vi "Main.vi"() -> ()   [LabVIEW 2014]
uses:
  bus_button.xctl
  VESA_Status.ctl
  Main_status.ctl
  <vilib>/Instr/_visa.llb/VISA Configure Serial Port (Instr).vi
  <vilib>/Instr/_visa.llb/VISA Serial Break (Instr).vi
panel:
  out "수신문자열(TEXT)":string
  in  "OUTPUT PULSE MODE":enum16{"uPPM(400Hz)", "PPM(40Hz)"}(ring)=enum."PPM(40Hz)"
  in  "서보제어":T1(array[cluster])=[{"리모트\nON/OFF"=TRUE, "PPM PULSE (ms)"=1500}, {"리모트\nON/OFF"=FALSE, "PPM PULSE (ms)"=1500}, {"리모트\nON/OFF"=FALSE, "PPM PULSE (ms)"=1500}] {"PPM PULSE (ms)" min=1000 max=2000 step=1 scale=1000.0..2000.0}
  out "전송문자열(TEXT)":string
  in  "UART":T3(xcontrol)={"VESA_Staus"=enum."DisConnect", "COM_Port"="COM3"}
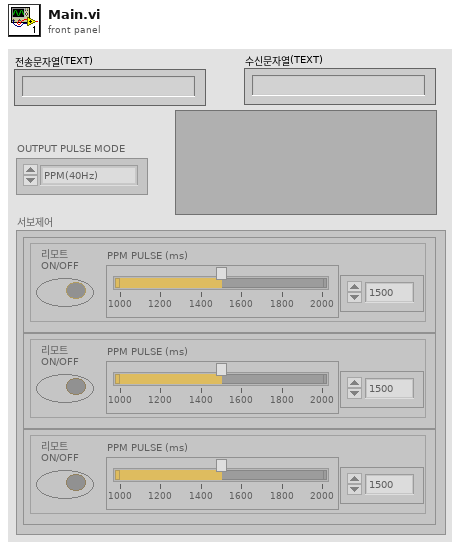
[diagram p1: front panel]
types:
  T1 = cluster{"리모트\nON/OFF":bool, "PPM PULSE (ms)":u16}[]
  T2 = typedef "bus_button.xctl/VESA_Status.ctl" = enum16{"Init", "Wait", "Connect", "DisConnect", "Idel", "Exit"}
  T3 = cluster{"VESA_Staus":T2, "COM_Port":refnum<visa-resource-name>}
  T4 = typedef "Main_status.ctl" = enum16{"Init", "Wait", "connect", "Idle", "disc", "Exit"}
  T5 = enum8{"Enabled", "Disabled", "Disabled and Grayed Out"}
  T6 = cluster{"리모트\nON/OFF":bool, "PPM PULSE (ms)":bool}[]
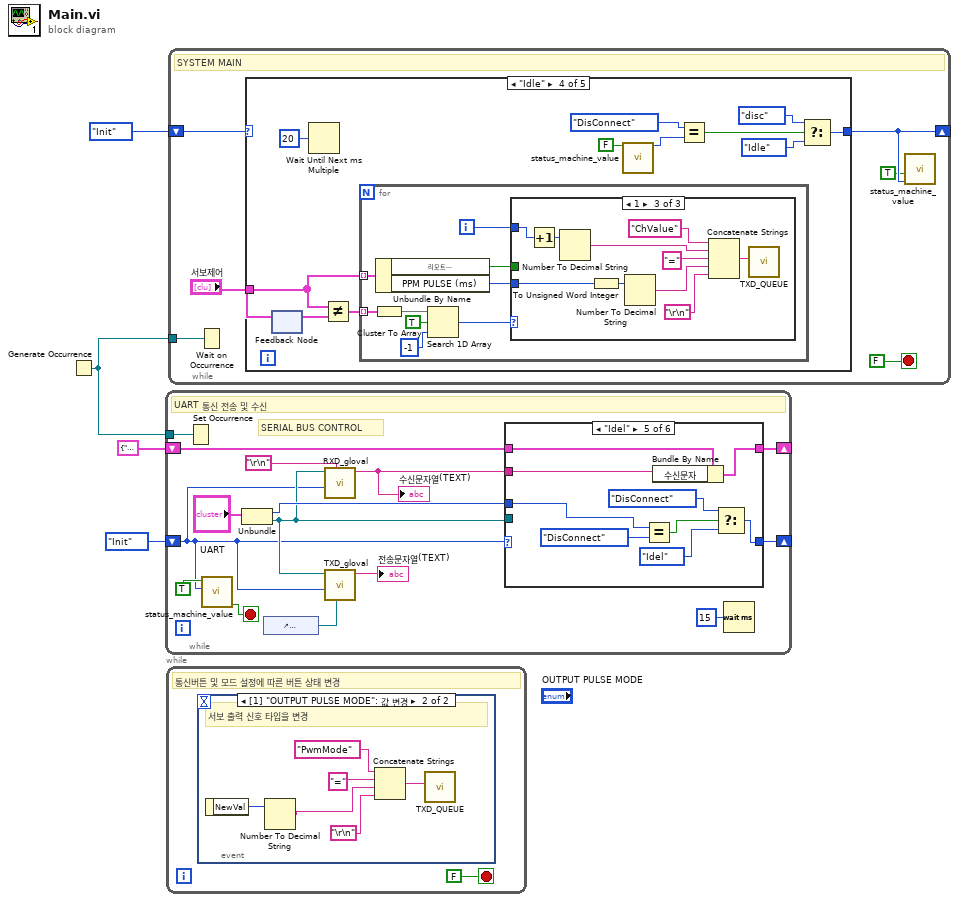
[diagram p0: block diagram]
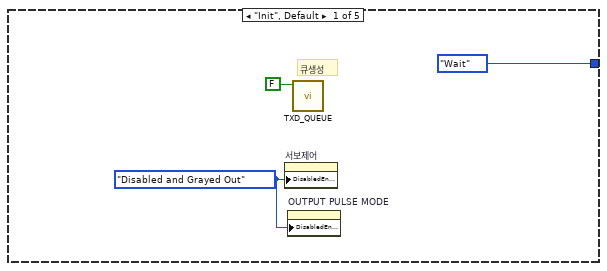
[diagram p2: hidden frame]
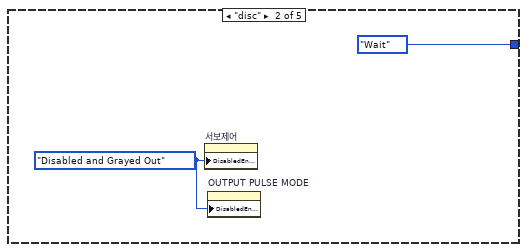
[diagram p3: hidden frame]
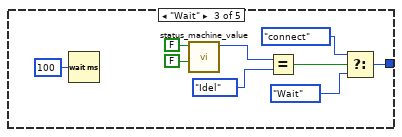
[diagram p4: hidden frame]
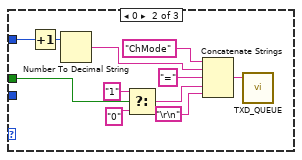
[diagram p6: hidden frame]
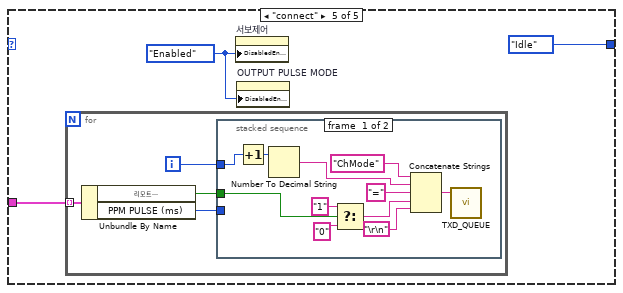
[diagram p7: hidden frame]
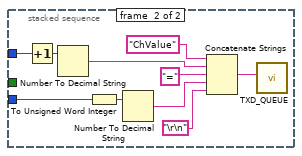
[diagram p8: hidden frame]
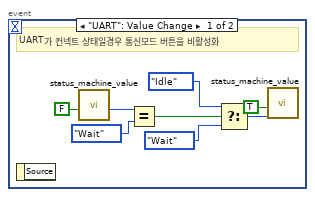
[diagram p9: hidden frame]
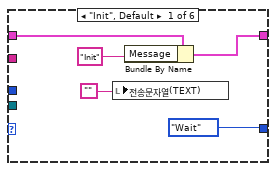
[diagram p10: hidden frame]
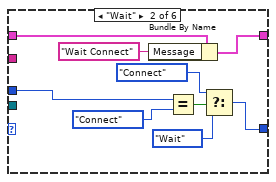
[diagram p11: hidden frame]
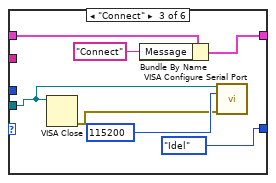
[diagram p12: hidden frame]
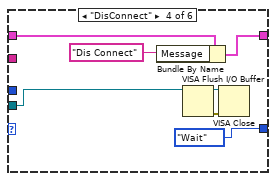
[diagram p13: hidden frame]
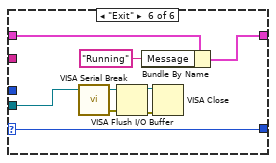
[diagram p14: hidden frame]
diagram:
  n1 = Generate Occurrence() -> (w1:refnum<k4>)
  n2 = while {
    shift-right: [w16] -> _
    shift-left: VESA_Status."Init" -> [w8]
    shift-right: [w18] -> _
    shift-left: cluster{"Message":string, "수신문자":string} {"Message"="", "수신문자"=""} -> [w17]
    tunnel: w1 -> [w11]
    stop <- w7 stop-if-true
    # "SERIAL BUS CONTROL"
    # "UART 통신 전송 및 수신"
    n3 = Set Occurrence(w11) -> ()
    n4 = call "status_machine_value.vi"("Vesa_Status_in"=w8, "vesa상태쓰기"=TRUE) -> ("Main Exit?"=w7:bool)  [unwired: 6 in, 3 out]
    n5 = Unbundle("UART") -> ("VESA_Staus"=w15:T2, "COM_Port"=w14:refnum<visa-resource-name>)
    n6 = control-ref of="전송문자열(TEXT)"() -> (w13:refnum<vi>)
    n7 = call "RXD_gloval.vi"("종료문자열"="\r\n", "Vesa_Status"=w8, "SERIAL.COM_Port"=w14) -> ("수신문자"=w5:string)  [unwired: 8 in]
    "수신문자열(TEXT)" <- w5
    n8 = call "TXD_gloval.vi"("전송문자열참조"=w13, "Vesa_Status"=w8, "SERIAL.COM_Port"=w14) -> ("전송문자열"=→"전송문자열(TEXT)":string)  [unwired: 7 in, 1 out]
    n9 = case shown="\"Idel\"" w8 {
      selector: w8 -> [_ _ _ _ _ w62]
      tunnel: w17 -> [w22 w31 w38 w45 w56 w63]
      tunnel: [w23 w32 w40 w46 w55 w64] -> w18
      tunnel: [VESA_Status."Wait" ("VESA_Staus") w25 VESA_Status."Idel" ("VESA_Staus") VESA_Status."Wait" ("VESA_Staus") w49 w62] -> w16
      tunnel: w14 -> [_ _ w34 w41 _ w57]
      tunnel: w15 -> [_ w26 _ _ w50 _]
      tunnel: w5 -> [_ _ _ _ w48 _]
      frame "Init", Default {
        n10 = local write "전송문자열(TEXT)"("") -> ()
        n11 = Bundle By Name(cluster=w22, "Message"="Init") -> (w23:cluster{"Message":string, "수신문자":string})
      }
      frame "Wait" {
        n12 = Bundle By Name(cluster=w31, "Message"="Wait Connect") -> (w32:cluster{"Message":string, "수신문자":string})
        n13 = Equal?(x=w26, y=VESA_Status."Connect" ("VESA_Staus")) -> (x = y?=w29:bool)
        n14 = Select(t=VESA_Status."Connect" ("VESA_Staus"), s=w29, f=VESA_Status."Wait") -> (s? t:f=w25:T2)
      }
      frame "Connect" {
        n15 = VISA Close(VISA resource name=w34) -> (error out=w35:errorcluster)  [unwired: 1 in]
        n16 = Bundle By Name(cluster=w38, "Message"="Connect") -> (w40:cluster{"Message":string, "수신문자":string})
        n17 = call-poly "VISA Configure Serial Port"("VISA resource name"=w34, "baud rate (9600)"=u32 115200, "error in (no error)"=w35) -> ()  [unwired: 11 in, 2 out]
      }
      frame "DisConnect" {
        n18 = Bundle By Name(cluster=w45, "Message"="Dis Connect") -> (w46:cluster{"Message":string, "수신문자":string})
        n19 = VISA Flush I/O Buffer(VISA resource name=w41) -> (VISA resource name out=w43:refnum<visa-resource-name>, error out=w42:errorcluster)  [unwired: 2 in]
        n20 = VISA Close(VISA resource name=w43, error in (no error)=w42) -> ()  [unwired: 1 out]
      }
      frame "Idel" {
        n21 = Equal?(x=w50, y=VESA_Status."DisConnect" ("VESA_Staus")) -> (x = y?=w53:bool)
        n22 = Bundle By Name(cluster=w56, "수신문자"=w48) -> (w55:cluster{"Message":string, "수신문자":string})
        n23 = Select(t=VESA_Status."DisConnect" ("VESA_Staus"), s=w53, f=VESA_Status."Idel") -> (s? t:f=w49:T2)
      }
      frame "Exit" {
        n24 = call-poly <vilib>:"VISA Serial Break.vi"("VISA resource name"=w57) -> ("error out"=w59:errorcluster, "VISA resource name out"=w58:refnum<visa-resource-name>)  [unwired: 3 in]
        n25 = VISA Flush I/O Buffer(VISA resource name=w58, error in (no error)=w59) -> (VISA resource name out=w60:refnum<visa-resource-name>, error out=w61:errorcluster)  [unwired: 1 in]
        n26 = Bundle By Name(cluster=w63, "Message"="Running") -> (w64:cluster{"Message":string, "수신문자":string})
        n27 = VISA Close(VISA resource name=w60, error in (no error)=w61) -> ()  [unwired: 1 out]
      }
    }
    n28 = Wait (ms)(milliseconds to wait=u32 15 ("대기 시간(ms)")) -> ()  [unwired: 1 out]
  }
  n29 = while {
    stop <- FALSE stop-if-true
    # "통신버튼 및 모드 설정에 따른 버튼 상태 변경"
    n30 = event shown="[1] \"OUTPUT PULSE MODE\": 값 변경" {
      selector: _ -> [_ _]
      dyn-events: _ -> [_ _]
      timeout: _ -> [_ _]
      event "UART": Value Change {
        # "UART가 컨넥트 상태일경우 통신모드 버튼을 비활성화"
        n31 = event-data() -> ()  [unwired: 1 in, 1 out]
        n32 = call "status_machine_value.vi"("Main상태쓰기"=FALSE) -> ("Main_Status"=w73:T4)  [unwired: 7 in, 3 out]
        n33 = Equal?(x=w73, y=Main_status."Wait") -> (x = y?=w67:bool)
        n34 = Select(t=Main_status."Idle" ("Main_Status_in"), s=w67, f=Main_status."Wait") -> (s? t:f=w68:T4)
        n35 = call "status_machine_value.vi"("Main_Status_in"=w68, "Main상태쓰기"=TRUE) -> ()  [unwired: 6 in, 4 out]
      }
      event "OUTPUT PULSE MODE": Value Change {
        # "서보 출력 신호 타입을 변경"
        n36 = event-data() -> ("NewVal"=w77:enum16{"uPPM(400Hz)", "PPM(40Hz)"})  [unwired: 1 in]
        n37 = Number To Decimal String(number=w77) -> (decimal integer string=w76:string)  [unwired: 1 in]
        n38 = Concatenate Strings("PwmMode", "=" ("문자열"), w76, "\r\n") -> (w80:string)
        n39 = call "TXD_QUEUE.vi"("송신문자"=w80) -> ()  [unwired: 9 in, 2 out]
      }
    }
  }
  n40 = while {
    shift-right: [w83] -> _
    shift-left: Main_status."Init" ("Main_Status") -> [w84]
    tunnel: w1 -> [w85]
    stop <- FALSE stop-if-true
    # "SYSTEM MAIN"
    n41 = Wait on Occurrence(2:w85) -> ()  [unwired: 2 in, 1 out]
    n42 = case shown="\"Idle\"" w84 {
      tunnel: [Main_status."Wait" ("f") Main_status."Wait" ("f") w100 w101 Main_status."Idle" ("f")] -> w83
      tunnel: "서보제어" -> [_ _ _ w107 w143]
      frame "Init", Default {
        w87 = T5."Disabled and Grayed Out" ("비활성화")
        # "큐생성"
        n43 = property on="서보제어" class="Arr (엄격한)"("DisabledEnum"=w87) -> ()  [unwired: 2 in, 2 out]
        n44 = property on="OUTPUT PULSE MODE" class="Enum (엄격한)"("DisabledEnum"=w87) -> ()  [unwired: 2 in, 2 out]
        n45 = call "TXD_QUEUE.vi"("전송?"=FALSE) -> ()  [unwired: 9 in, 2 out]
      }
      frame "disc" {
        w90 = T5."Disabled and Grayed Out" ("비활성화")
        n46 = property on="서보제어" class="Arr (엄격한)"("DisabledEnum"=w90) -> ()  [unwired: 2 in, 2 out]
        n47 = property on="OUTPUT PULSE MODE" class="Enum (엄격한)"("DisabledEnum"=w90) -> ()  [unwired: 2 in, 2 out]
      }
      frame "Wait" {
        n48 = Wait (ms)(milliseconds to wait=u32 100 ("대기 시간(ms)")) -> ()  [unwired: 1 out]
        n49 = call "status_machine_value.vi"("Main상태쓰기"=FALSE, "vesa상태쓰기"=FALSE) -> ("Vesa_Status"=w98:T2)  [unwired: 6 in, 3 out]
        n50 = Equal?(x=w98, y=VESA_Status."Idel") -> (x = y?=w94:bool)
        n51 = Select(t=Main_status."connect" ("Main_Status"), s=w94, f=Main_status."Wait") -> (s? t:f=w100:T4)
      }
      frame "Idle" {
        n52 = feedback #1() -> (w109:T1)  [unwired: 1 in]
        n53 = feedback-in #1(w107) -> ()
        n54 = Wait Until Next ms Multiple(millisecond multiple=u32 20 ("ms 배수")) -> ()  [unwired: 1 out]
        n55 = Not Equal?(x=w107, y=w109) -> (x != y?=w108:T6)
        n56 = for {
          tunnel: w108 -> [w115] mode=indexing
          tunnel: w107 -> [w114] mode=indexing
          i -> [w116]
          n57 = Cluster To Array(cluster=w115) -> (array=w120:bool[])
          n58 = Unbundle By Name(w114) -> ("리모트\nON/OFF"=w113:bool, "PPM PULSE (ms)"=w112:u16)
          n59 = Search 1D Array(1D array=w120, element=TRUE ("원소"), start index (0)=-1 ("시작 인덱스(0)")) -> (index of element=w117:i32)
          n60 = case shown="1" w117 {
            tunnel: w116 -> [_ w123 w134]
            tunnel: w113 -> [_ w121 _]
            tunnel: w112 -> [_ _ w133]
            frame -1, Default {
            }
            frame 0 {
              n61 = Increment(x=w123) -> (x+1=w124:i32)
              n62 = Number To Decimal String(number=w124) -> (decimal integer string=w122:string)  [unwired: 1 in]
              n63 = Select(t="1", s=w121, f="0") -> (s? t:f=w128:string)
              n64 = Concatenate Strings("ChMode", w122, "=" ("문자열"), w128, "\r\n") -> (w127:string)
              n65 = call "TXD_QUEUE.vi"("송신문자"=w127) -> ()  [unwired: 9 in, 2 out]
            }
            frame 1 {
              n66 = Increment(x=w134) -> (x+1=w139:i32)
              n67 = Number To Decimal String(number=w139) -> (decimal integer string=w141:string)  [unwired: 1 in]
              n68 = To Unsigned Word Integer(number=w133) -> (unsigned 16bit integer=w138:u16)
              n69 = Number To Decimal String(number=w138) -> (decimal integer string=w136:string)  [unwired: 1 in]
              n70 = Concatenate Strings("ChValue", w141, "=" ("문자열"), w136, "\r\n") -> (w132:string)
              n71 = call "TXD_QUEUE.vi"("송신문자"=w132) -> ()  [unwired: 9 in, 2 out]
            }
          }
        }
        n72 = call "status_machine_value.vi"("vesa상태쓰기"=FALSE) -> ("Vesa_Status"=w105:T2)  [unwired: 7 in, 3 out]
        n73 = Equal?(x=VESA_Status."DisConnect" ("Vesa_Status"), y=w105) -> (x = y?=w104:bool)
        n74 = Select(t=Main_status."disc" ("Main_Status"), s=w104, f=Main_status."Idle") -> (s? t:f=w101:T4)
      }
      frame "connect" {
        w142 = T5."Enabled" ("비활성화")
        n75 = for {
          tunnel: w143 -> [w147] mode=indexing
          i -> [w148]
          n76 = Unbundle By Name(w147) -> ("리모트\nON/OFF"=w146:bool, "PPM PULSE (ms)"=w145:u16)
          n77 = stacked-sequence {
            tunnel: w148 -> [w151 w162]
            tunnel: w146 -> [w149 _]
            tunnel: w145 -> [_ w161]
            frame #0 {
              n78 = Increment(x=w151) -> (x+1=w152:i32)
              n79 = Number To Decimal String(number=w152) -> (decimal integer string=w150:string)  [unwired: 1 in]
              n80 = Select(t="1", s=w149, f="0") -> (s? t:f=w156:string)
              n81 = Concatenate Strings("ChMode", w150, "=" ("문자열"), w156, "\r\n") -> (w155:string)
              n82 = call "TXD_QUEUE.vi"("송신문자"=w155) -> ()  [unwired: 9 in, 2 out]
            }
            frame #1 {
              n83 = Increment(x=w162) -> (x+1=w167:i32)
              n84 = Number To Decimal String(number=w167) -> (decimal integer string=w169:string)  [unwired: 1 in]
              n85 = To Unsigned Word Integer(number=w161) -> (unsigned 16bit integer=w166:u16)
              n86 = Number To Decimal String(number=w166) -> (decimal integer string=w164:string)  [unwired: 1 in]
              n87 = Concatenate Strings("ChValue", w169, "=" ("문자열"), w164, "\r\n") -> (w160:string)
              n88 = call "TXD_QUEUE.vi"("송신문자"=w160) -> ()  [unwired: 9 in, 2 out]
            }
          }
        }
        n89 = property on="서보제어" class="Arr (엄격한)"("DisabledEnum"=w142) -> ()  [unwired: 2 in, 2 out]
        n90 = property on="OUTPUT PULSE MODE" class="Enum (엄격한)"("DisabledEnum"=w142) -> ()  [unwired: 2 in, 2 out]
      }
    }
    n91 = call "status_machine_value.vi"("Main_Status_in"=w83, "Main상태쓰기"=TRUE) -> ()  [unwired: 6 in, 4 out]
  }
